vi "Log.vi"(9 "Log Packet":T1, 10 "Message":string="Log Entry", 11 "LoggerReference in":refnum<class "LoggerReference.lvclass">) -> (0 "error out":errorcluster, 3 "LoggerReference out":refnum<class "LoggerReference.lvclass">)   [LabVIEW 2017, in "Composed Log.lvlib" / "LoggerReference.lvclass"]
uses:
  <vilib>/gpm_packages/@cs/event-logger/Source/Composed Log/LoggerReference/LoggerReference.lvclass
  <vilib>/gpm_packages/@cs/event-logger/Source/Composed Log/Types/Log Packet.ctl
  <vilib>/gpm_packages/@cs/event-logger/Source/Composed Log/Types/Log Level.ctl
  <vilib>/gpm_packages/@cs/event-logger/Source/Composed Log/LoggerReference/LoggerReference.lvclass/LoggerReference.ctl
  <vilib>/gpm_packages/@cs/event-logger/Source/Composed Log/Types/MessageCluster.ctl
  <vilib>/gpm_packages/@cs/event-logger/Source/Composed Log/Composed Log.lvlib
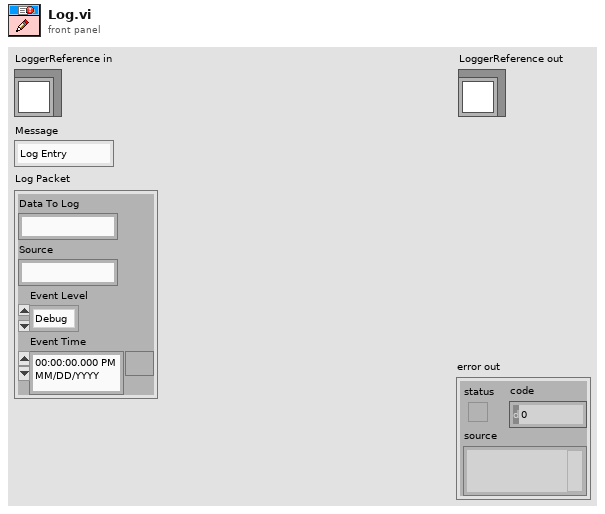
[diagram p1: front panel]
types:
  T1 = typedef "Composed Log.lvlib/Log Packet.ctl" = cluster{"Data To Log":string, "Source":string, "Event Level":T2, "Event Time":timestamp}
  T2 = typedef "Composed Log.lvlib/Log Level.ctl" = enum16{"Debug", "Info", "Warning", "Error", "Critical"}
  T3 = typedef "Composed Log.lvlib/MessageCluster.ctl" = cluster{"Message":string, "Data":variant}
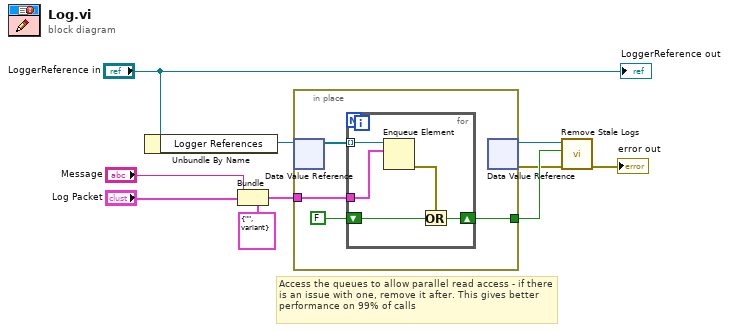
[diagram p0: block diagram]
diagram:
  # "Access the queues to allow parallel read access - if there is an issue with one, remove it after. This gives better performance on 99% of calls"
  n1 = Unbundle By Name("LoggerReference in") -> ("Logger References"=w8:refnum<data-value>)
  n2 = Bundle(cluster=T3 {"Message"="", "Data"=variant} ("element"), "Message"="Message", "Data"="Log Packet") -> (w1:T3)
  n3 = in-place {
    in-place-border: [w12] -> w6
    in-place-border: w1 -> [w11]
    n4 = in-place-dvr #1(w8) -> (w14:refnum<queue>[])  [unwired: 1 out]
    n5 = for {
      shift-right: [w19] -> w12
      shift-left: FALSE -> [w18]
      tunnel: w14 -> [w16] mode=indexing
      tunnel: w11 -> [w15]
      n6 = Enqueue Element(queue=w16, element=w15) -> (error out=w17:errorcluster)  [unwired: 2 in, 2 out]
      n7 = Or(x=w17, y=w18) -> (x .or. y?=w19:bool)
    }
    n8 = in-place-dvr #1() -> (w7:refnum<data-value>, w5:errorcluster)  [unwired: 1 in]
  }
  n9 = call <vilib>:"Remove Stale Logs.vi"("error in (no error)"=w5, "Bad Log?"=w6, "Aggregate Logs In"=w7) -> ("error out"=→"error out":errorcluster)  [unwired: 7 in, 1 out]
  "LoggerReference out" <- "LoggerReference in"
